vi "Process.vi"(8 "error in":errorcluster, 11 "Instrument.Transport in":refnum<class "Inst.Transport.lvclass">) -> (0 "error out":errorcluster, 3 "Instrument.Transport out":refnum<class "Inst.Transport.lvclass">)   [LabVIEW 2019, in "Inst.Transport.lvclass"]
doc: "---------------------------------------------------------------\nJKI State Machine Objects™\nhttp://jki.net/state-machine-objects/\nCopyright (C) 2005-2015, JKI <info@jki.net>\nALL RIGHTS RESERVED"
uses:
  Inst.Transport.lvclass
  <userlib>/LevyLab/Instrument Framework/Instrument/Instrument.lvclass
  <userlib>/LevyLab/RemoteControl/RemoteControl/Typedefs/Message--Cluster.ctl
  <userlib>/LevyLab/RemoteControl/RemoteControl/RemoteControl.lvclass
  Typedefs/PrivateEvents--MessageToProcess.ctl
  <userlib>/LevyLab/Debug/Debug.lvlib
  <vilib>/JKI/JKI SMO/SMO/SMO.lvclass
  <userlib>/LevyLab/Instrument Framework/Instrument Types/SCPI/Instrument.SCPI.lvclass
  <userlib>/LevyLab/Transport/Control Experiment/Control Experiment.lvclass
  <userlib>/LevyLab/Transport/Transport/Transport.lvclass
  <vilib>/platform/TimedLoop/XDataNode/XDataNode.xnode
  <vilib>/Platform/TimedLoop/XDataNode/timing_clust.ctl
  <vilib>/Platform/TimedLoop/XDataNode/XDNodeRunTimeDep.lvlib
  <vilib>/Platform/TimedLoop/XDataNode/wakeup.ctl
  <vilib>/Platform/TimedLoop/XDataNode/nitl_modes.ctl
  <userlib>/LevyLab/Lockin-Multichannel/Instrument.DAQ/Typedefs/Sweep.Pattern--Enum.ctl
  <userlib>/LevyLab/Lockin-Multichannel/Instrument.DAQ/Instrument.DAQ.lvclass
  <userlib>/LevyLab/Lockin-Multichannel/Instrument.DAQ/Typedefs/Sweep.Channel--Cluster.ctl
  <userlib>/LevyLab/Lockin-Multichannel/Instrument.DAQ/Typedefs/Sweep.Channel--Cluster--Array.ctl
  <userlib>/LevyLab/Transport/Transport/Typedefs/Lockin_Sweep JSON--Cluster.ctl
  <userlib>/LevyLab/Instrument Framework/Instrument/API/Instrument.sendMessageToProcess (variant).vi
  C:/Program Files (x86)/National Instruments/LabVIEW 2019/user.lib/LevyLab/Instrument Framework/Instrument Types/SCPI/Instrument.SCPI.lvclass
  C:/Program Files (x86)/National Instruments/LabVIEW 2019/user.lib/LevyLab/Instrument Framework/Instrument/Instrument.lvclass
  C:/Program Files (x86)/National Instruments/LabVIEW 2019/vi.lib/JKI/JKI SMO/SMO/SMO.lvclass
panel:
  in  "stop 2":bool
  in  "stop":bool
  out "Calling VI":string
  out "Experiment Folder":string
  out "Comments":string
  out "TDMS Params":cluster{"Key":string, "Value":dbl}[](array[cluster])
  out "Status":string
  out "State History":string
  # "Instrument.Framework-Template"
  # "Framework-Template"
  # "For instructions on how to use the JKI State Machine Objects, examples and video tutorials, visit:\nhttp://jki.net/state-machine-objects/\n\nJKI State Machine Objects™\nhttp://jki.net/state-machine-objects/\nCopyright (C) 2005-2015, JKI <info@jki.net>\nALL RIGHTS RESERVED"
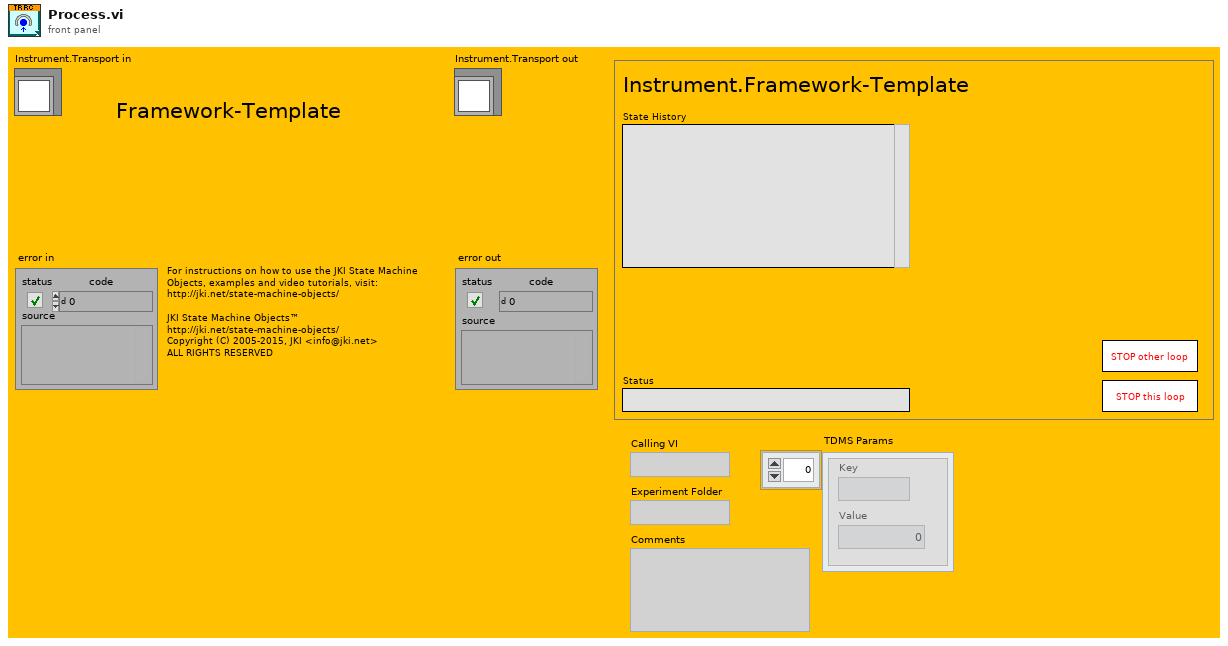
[diagram p1: front panel]
types:
  T1 = typedef "Transport.lvclass/Lockin_Sweep JSON--Cluster.ctl" = cluster{"Sweep Time (s)":dbl, "Initial Wait (s)":dbl, "Return to Start":bool, "Sweep Channels":T2, "Sweep Tables":cluster{"Ch":i32, "Table":dbl[]}[]}
  T2 = typedef "Instrument.Lockin.lvlib/Instrument.DAQ.lvclass/Sweep.Channel--Cluster--Array.ctl" = T3[]
  T3 = typedef "Instrument.Lockin.lvlib/Instrument.DAQ.lvclass/Sweep.Channel--Cluster.ctl" = cluster{"Enable?":bool, "Channel":u16, "Start":dbl, "End":dbl, "Pattern":T4, "Table":dbl[]}
  T4 = typedef "Instrument.Lockin.lvlib/Instrument.DAQ.lvclass/Sweep.Pattern--Enum.ctl" = enum16{"Ramp /", "Ramp /\\", "Smooth Ramp _/", "Smooth Ramp _/\\_", "Table"}
  T5 = enum32{"invalid app kind", "Development System", "Run Time System", "Student Edition", "Embedded LabVIEW", "Evaluation", "Custom"}
  T6 = enum32{"Invalid", "Standard", "Closed", "Hidden", "Minimized", "Maximized"}
  T7 = typedef "RemoteControl.lvlib/RemoteControl.lvclass/Message--Cluster.ctl" = cluster{"Command":string, "Data":variant, "ID":string}
  T8 = typedef "Inst.Transport.lvclass/PrivateEvents--MessageToProcess.ctl" = cluster{"Message":T7}
  T9 = cluster{"Core":cluster{"Current VI Reference":refnum<vi>, "Close Panel on Exit?":bool, "Last Error":cluster{"error":errorcluster, "previous state":string, "remaining states":string}, "Shutdown?":bool}, "SelfRef":refnum<class "Inst.Transport.lvclass">, "HAL":refnum<class "HAL.lvclass">, "Running Step":i32, "sequence":string[], "MessageToProcess":T8, "UI Behavior":string, "wait":u32}
  T10 = cluster{"Current VI Reference":refnum<vi>, "Close Panel on Exit?":bool, "Last Error":cluster{"error":errorcluster, "previous state":string, "remaining states":string}, "Shutdown?":bool}
  T11 = typedef "Debug.lvlib/Attribute.Debug.lvclass/DebugBehavior.ctl" = enum16{"Normal", "Debug"}
  T12 = typedef "SMO.lvclass/Protected Events.ctl" = cluster{"StopProcesses":refnum<user-event>, "AbortProcesses":refnum<user-event>, "Config Changed":refnum<user-event>, "Dependency":refnum<user-event>}
  T13 = typedef "Inst.Transport.lvclass/Inst.Transport.getAll--Cluster.ctl" = cluster{"Levy 1":dbl, "Logger SMO":dbl, "SMO Boolean":bool, "SMO String":string}
  T14 = typedef "XDNodeRunTimeDep.lvlib/timing_clust.ctl" = cluster{"Expected End [f-1]":u64, "Actual End [f-1]":u64, "Finished Late? [f-1]":bool, "Expected End [i-1]":u64, "Actual End [i-1]":u64, "Finished Late? [i-1]":bool, "Expected Start [i]":u64, "Actual Start [i]":u64, "Expected Start [f]":u64, "Actual Start [f]":u64, "Source Name":string, "Structure Name":string, "Period":i64, "Deadline":i64, "Offset":i64, "Start":i64, "Priority":i32, "Timeout":i32, "Mode":T15, "Wakeup Reason":T16, "Error":errorcluster, "Source Type":string, "Secondary Source Type":string, "Global End Time":u64, "Global Start Time":u64, "Frame Duration":u64, "Iteration Duration":u64, "Assigned CPU":i32, "I/O Scan Engine Mode":u32}
  T15 = typedef "XDNodeRunTimeDep.lvlib/nitl_modes.ctl" = enum32{"No Change", "Process missed periods, maintain original phase", "Discard missed periods, maintain original phase", "Process missed periods, ignore original phase", "Discard missed periods, ignore original phase"}
  T16 = typedef "XDNodeRunTimeDep.lvlib/wakeup.ctl" = enum32{"Normal", "Aborted", "Asynchronous wakeup", "Timing source error", "Timed loop error", "Timeout"}
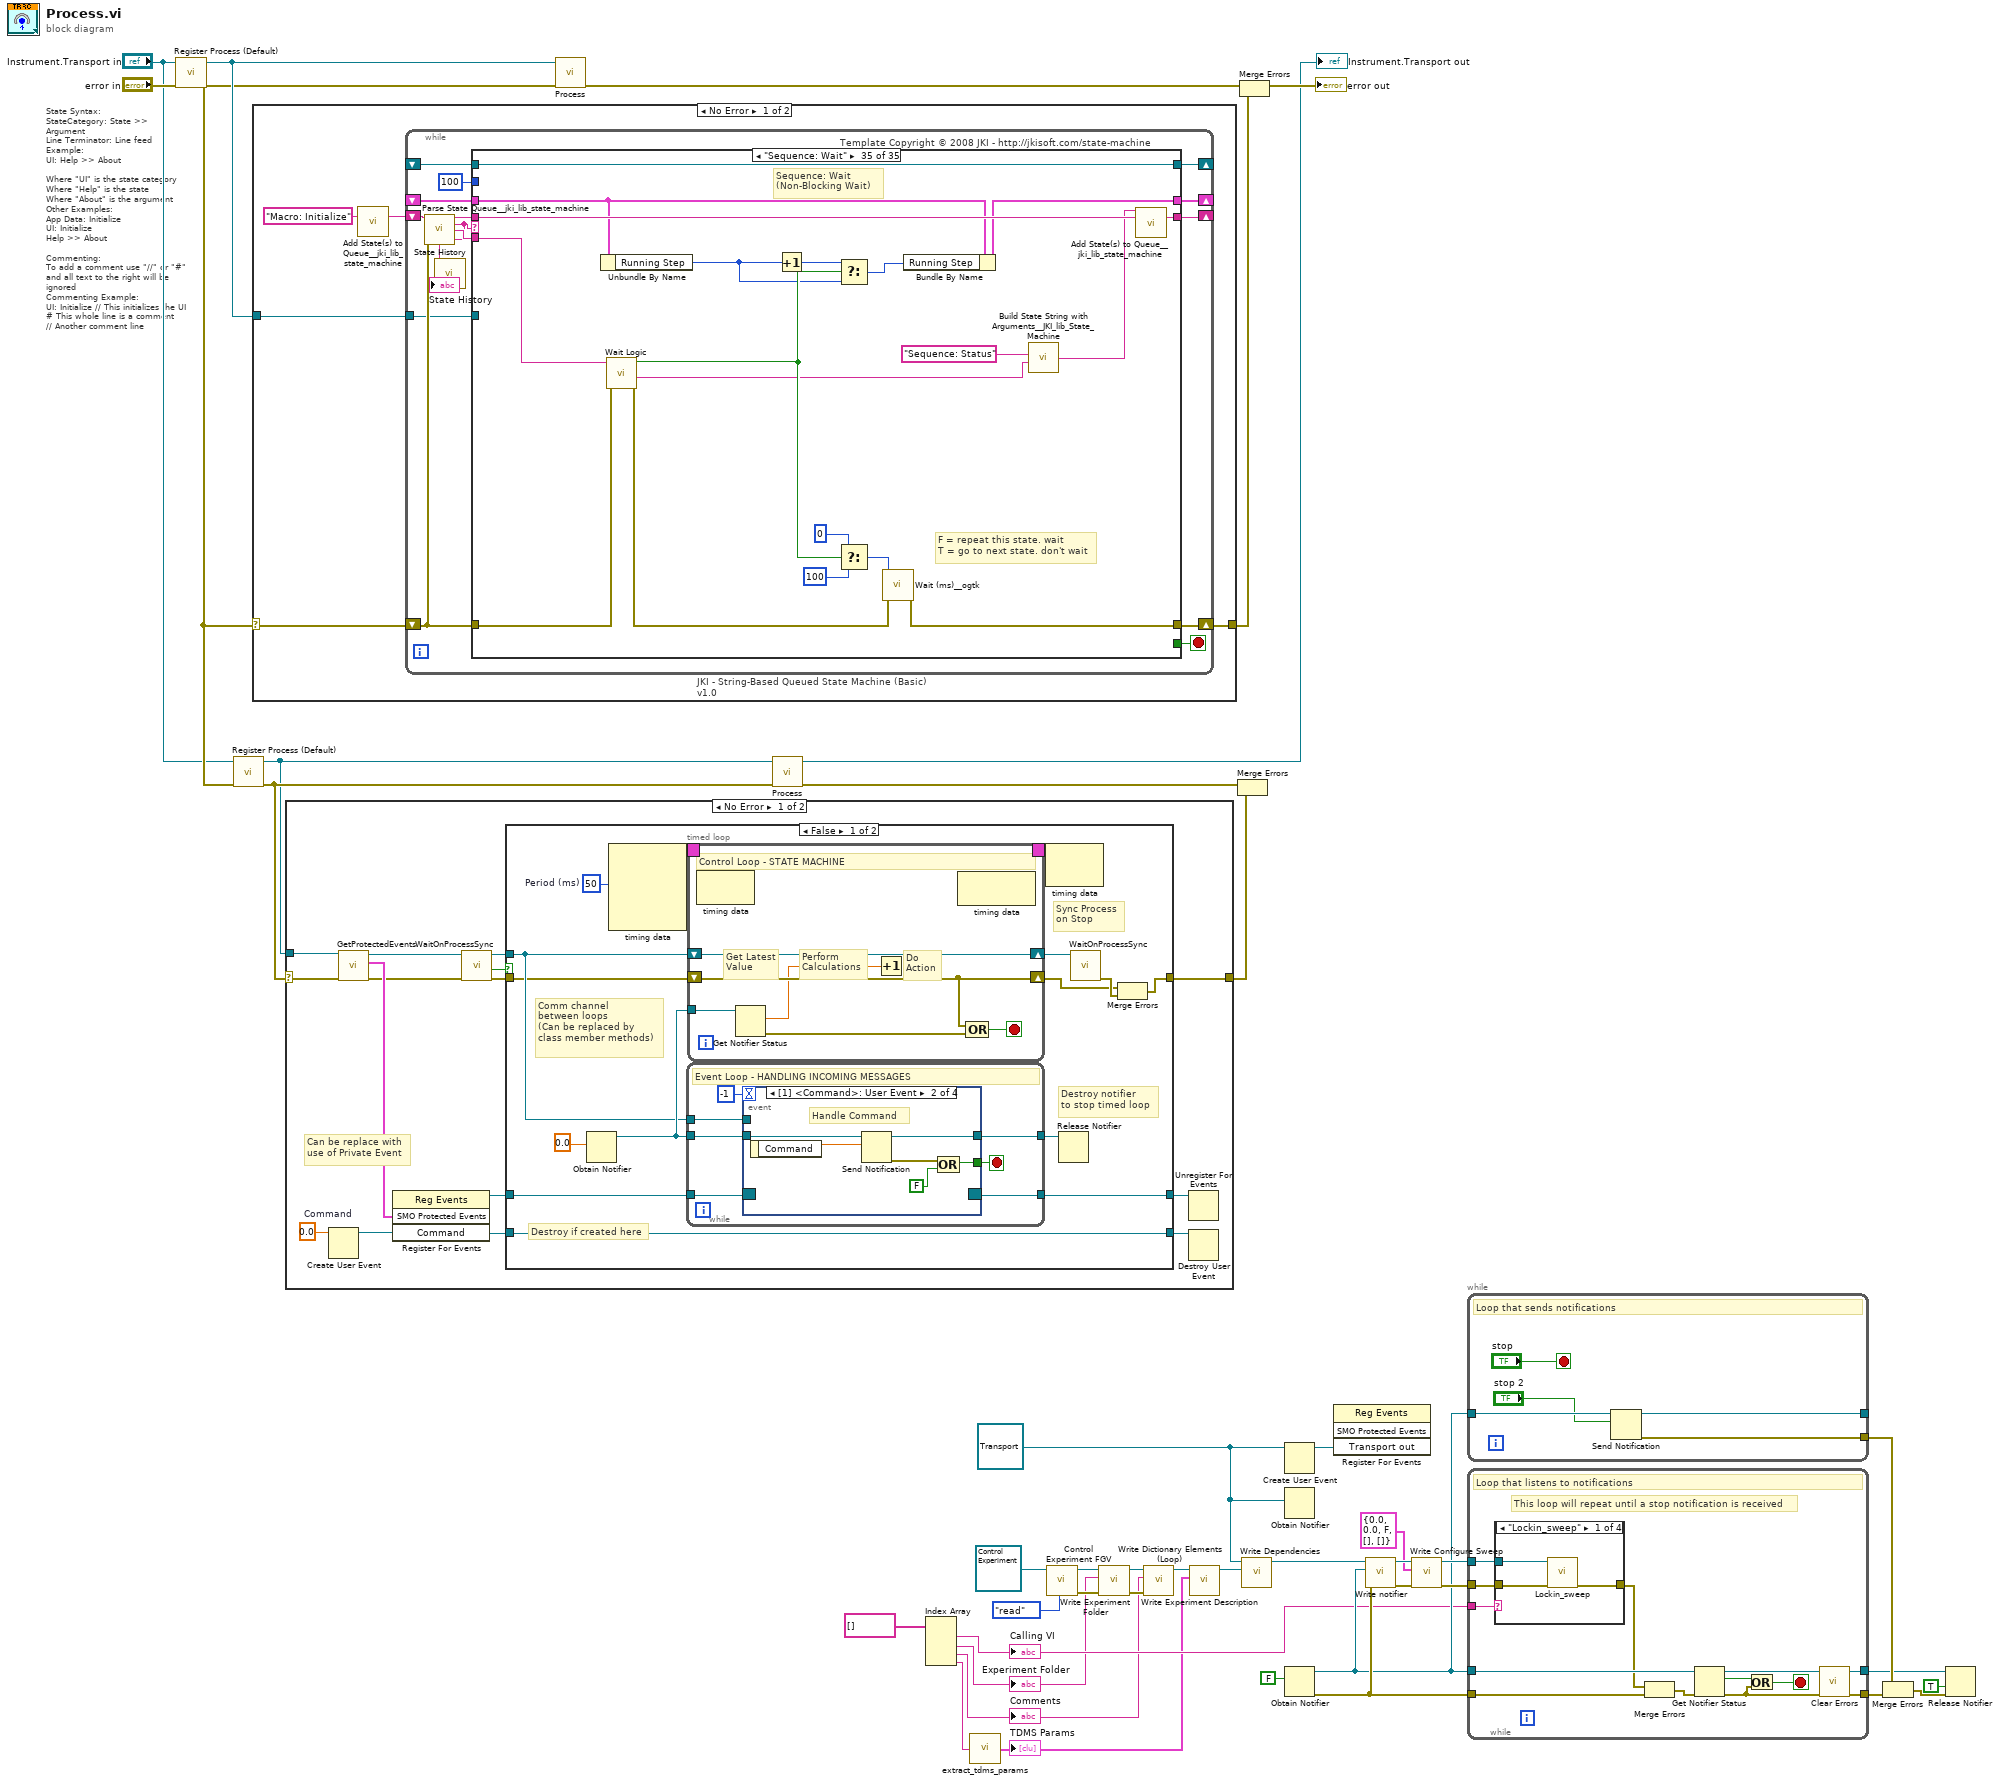
[diagram p0: block diagram]
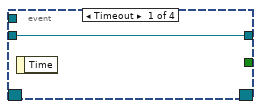
[diagram p2: hidden frame]
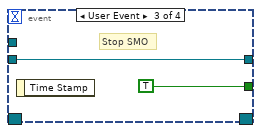
[diagram p3: hidden frame]
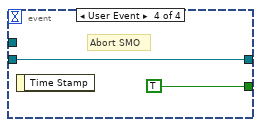
[diagram p4: hidden frame]
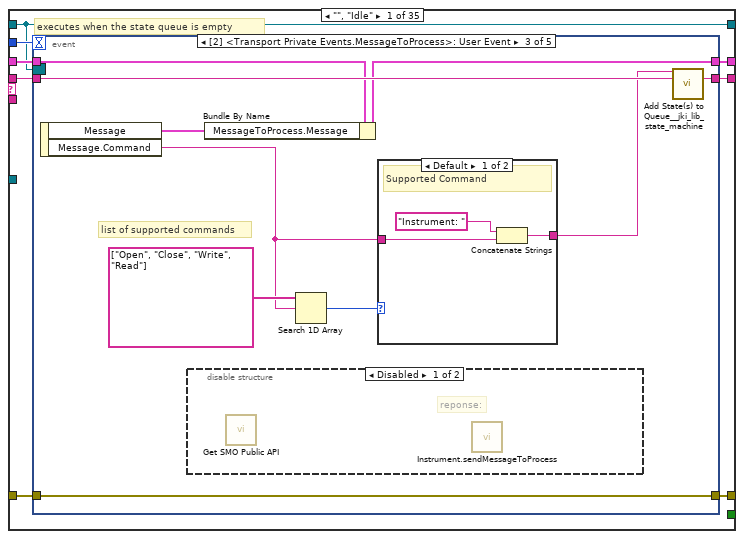
[diagram p7: hidden frame]
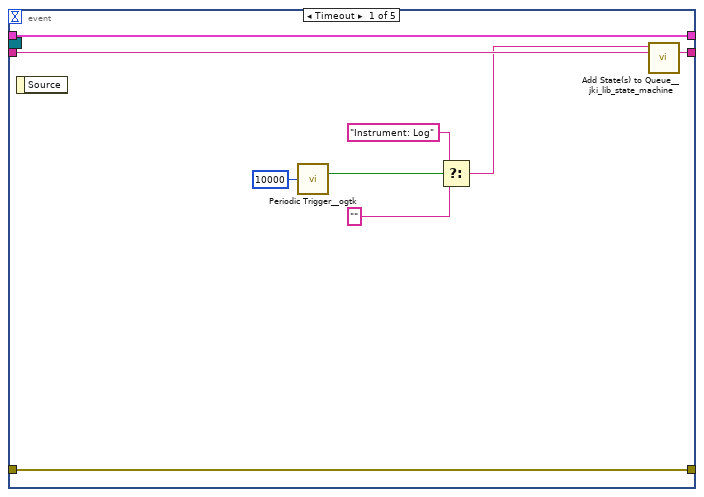
[diagram p8: hidden frame]
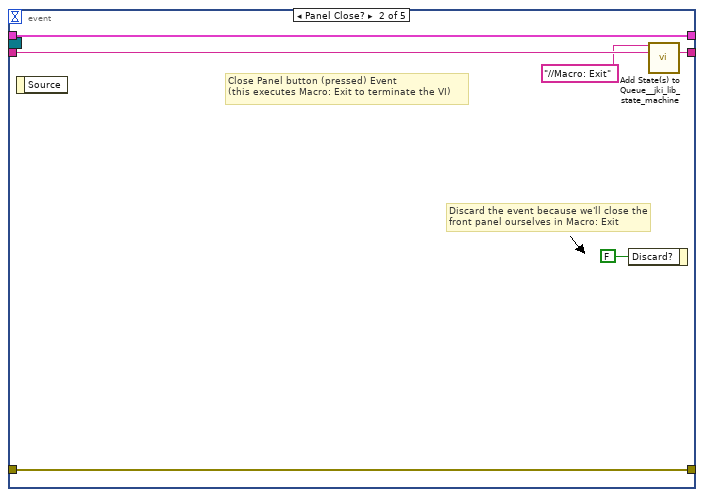
[diagram p9: hidden frame]
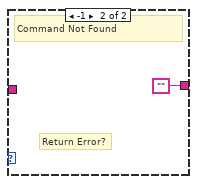
[diagram p11: hidden frame]
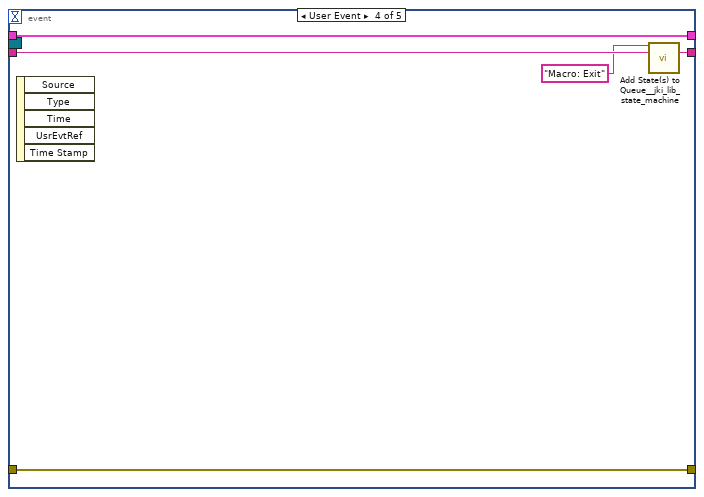
[diagram p12: hidden frame]
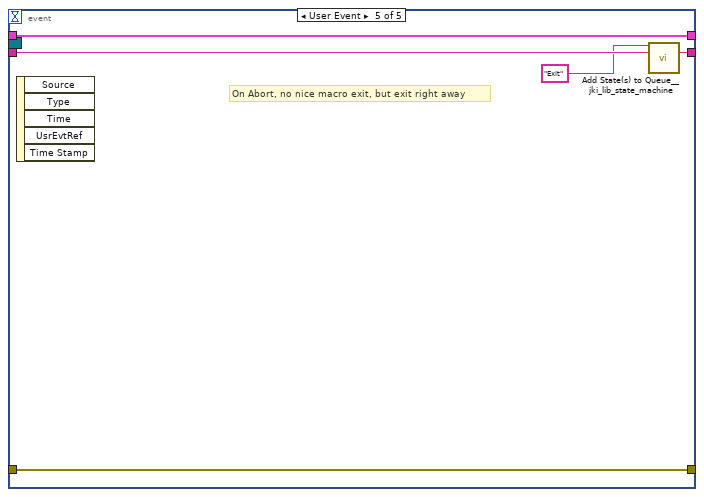
[diagram p13: hidden frame]
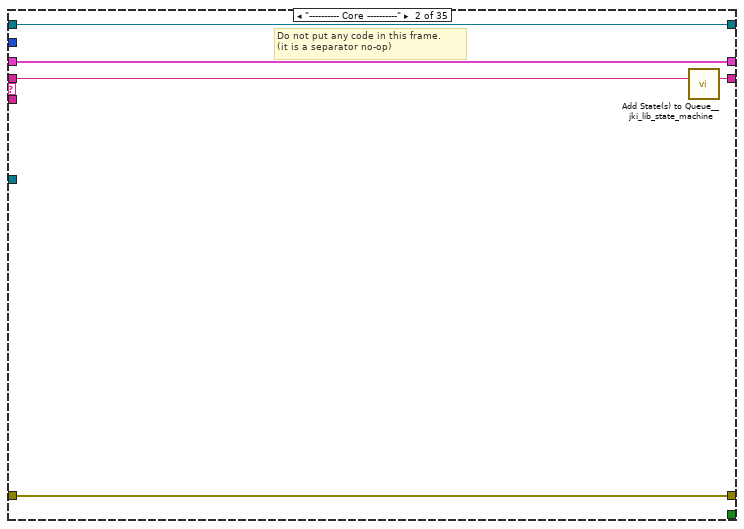
[diagram p14: hidden frame]
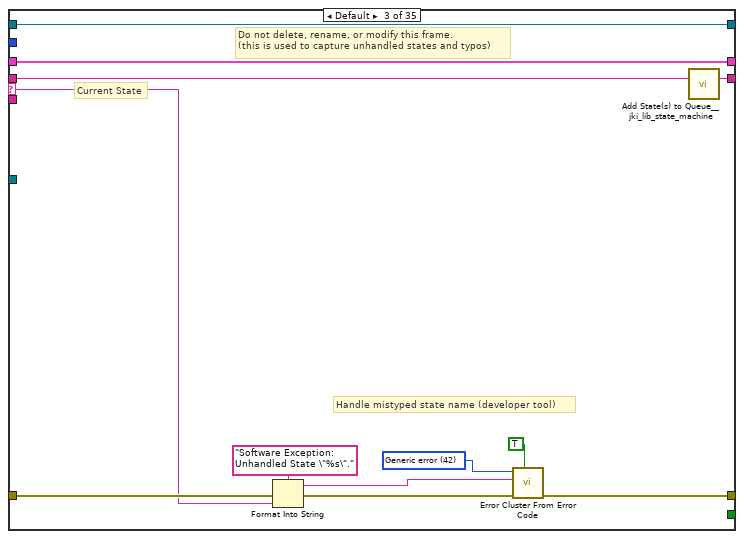
[diagram p15: hidden frame]
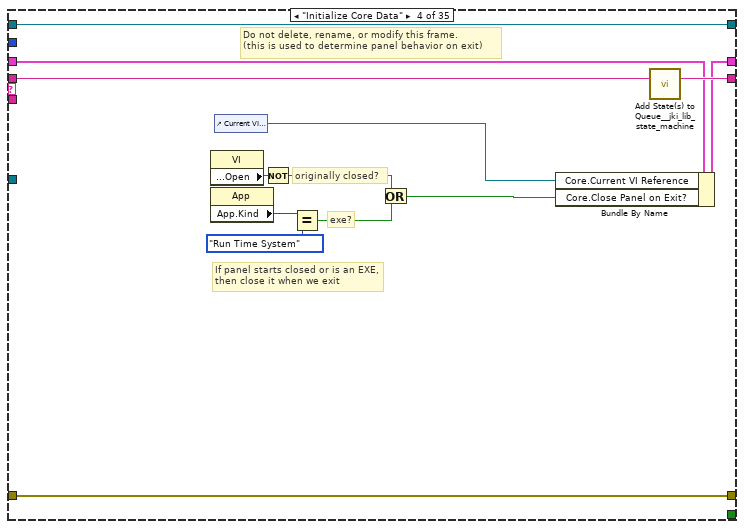
[diagram p16: hidden frame]
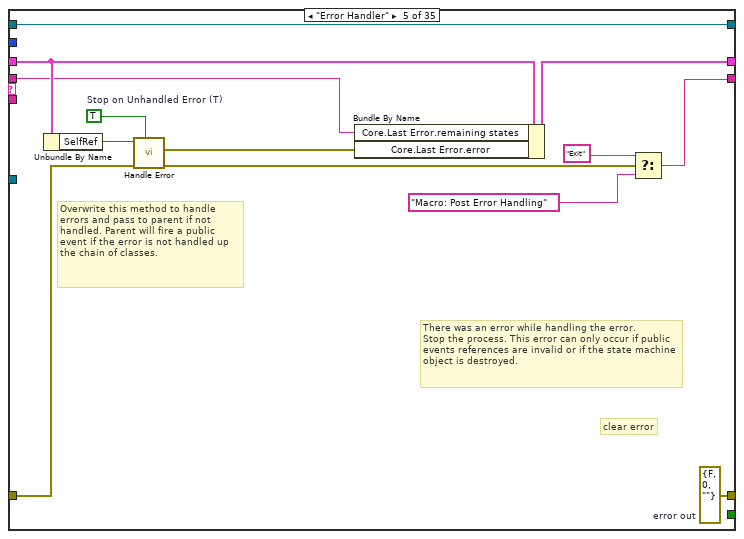
[diagram p17: hidden frame]
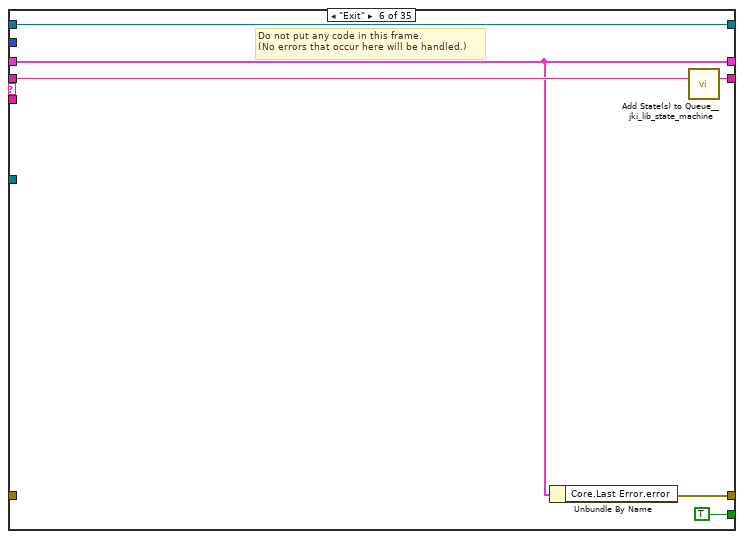
[diagram p18: hidden frame]
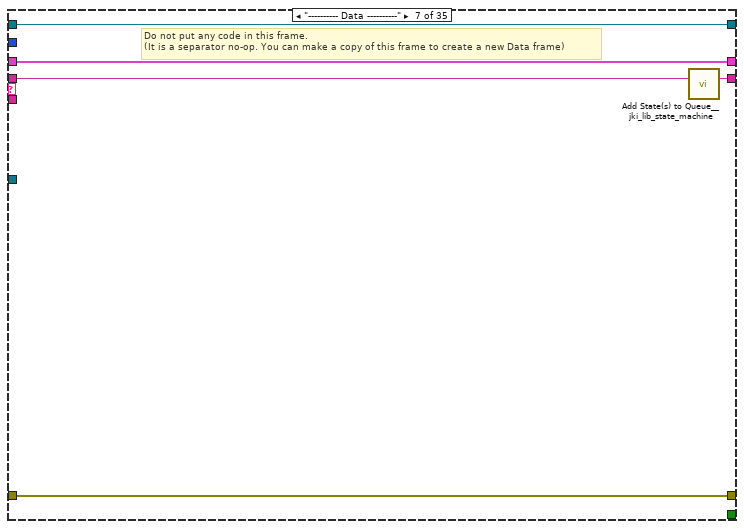
[diagram p19: hidden frame]
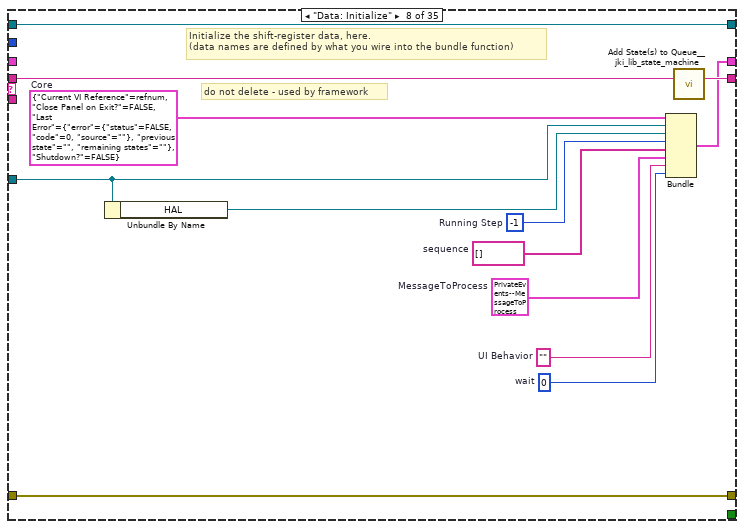
[diagram p20: hidden frame]
diagram:
  w2 = refnum<class "Transport.lvclass"> refnum ("Transport out")
  # "State Syntax:\nStateCategory: State >> Argument\nLine Terminator: Line feed\nExample:\nUI: Help >> About\n\nWhere \"UI\" is the state category\nWhere \"Help\" is the state\nWhere \"About\" is the argument\nOther Examples:\nApp Data: Initialize\nUI: Initialize\nHelp >> About\n\nCommenting:\nTo add a comment use \"//\" or \"#\" and all text to the right will be ignored\nCommenting Example:\nUI: Initialize // This initializes the UI\n# This whole line is a comment\n// Another comment line"
  n1 = call <vilib>:"Register Process (Default).vi"("error in (no error)"="error in", "SMO"="Instrument.Transport in") -> ("error out"=w33:errorcluster, "SelfRef"=w40:refnum<class "Inst.Transport.lvclass">)  [unwired: 8 in]
  n2 = call <vilib>:"Register Process (Default).vi"("error in (no error)"=w33, "SMO"="Instrument.Transport in") -> ("error out"=w37:errorcluster, "SelfRef"=w36:refnum<class "Inst.Transport.lvclass">)  [unwired: 8 in]
  n3 = case shown="No Error" w33 {
    selector: w33 -> [w44 w486]
    tunnel: w40 -> [w45 _]
    tunnel: [w43 w486] -> w38
    frame No Error {
      n4 = call <vilib>:"Add State(s) to Queue__jki_lib_state_machine.vi"("State(s) in (\"\")"="Macro: Initialize") -> ("States Out"=w47:string)  [unwired: 14 in]
      n5 = while "JKI - String-Based Queued State Machine (Basic) v1.0" {
        shift-right: [w56] -> _
        shift-left: _ -> [w55]
        shift-right: [w59] -> w43
        shift-left: w44 -> [w53]
        shift-right: [w58] -> _
        shift-left: w47 -> [w60]
        tunnel: w45 -> [w52]
        shift-right: [w51] -> _
        shift-left: _ -> [w50]
        stop <- w57 stop-if-true
        # "Template Copyright © 2008 JKI - http://jkisoft.com/state-machine"
        n6 = call <vilib>:"Parse State Queue__jki_lib_state_machine.vi"("State Queue"=w60, "Error In (no error)"=w53) -> ("Remaining States"=w62:string, "Current State"=w49:string, "Arguments"=w61:string)  [unwired: 11 in]
        n7 = call <userlib>:"State History.vi"("Current State"=w49) -> ("History"=→"State History":string)  [unwired: 10 in]
        n8 = case shown="\"Sequence: Wait\"" w49 {
          selector: w49 -> [_ _ w116 _ _ _ _ _ _ _ _ _ _ _ _ _ _ _ _ _ _ _ _ _ _ _ _ _ _ _ _ _ _ _ _]
          tunnel: w62 -> [w70 w114 w120 w139 w144 w158 w163 w176 w183 w188 w195 w204 w211 w227 w259 w268 w280 w301 w316 w338 w343 w354 w359 w372 w378 w386 w395 w404 w414 w423 w435 w455 w460 w466 w485]
          tunnel: w61 -> [_ _ _ _ _ _ _ _ _ _ _ w196 w205 w221 _ _ _ _ _ _ _ _ _ _ _ _ _ _ _ _ _ _ _ w461 w469]
          tunnel: w55 -> [w68 w111 w118 w130 w148 w154 w160 _ w178 w185 w193 w201 w209 w223 w256 w265 w270 w291 w305 w323 w340 w351 w356 w365 w376 w381 w391 w400 w410 w419 w431 w451 w456 w462 w475]
          tunnel: [w67 w112 w122 w136 w149 w153 w161 w166 w179 w186 w190 w202 w206 w224 w257 w260 w278 w299 w304 w326 w341 w345 w357 w368 w374 w383 w387 w399 w409 w418 w426 w449 w457 w463 w477] -> w59
          tunnel: w53 -> [w66 w112 w121 w136 w150 _ w161 w166 w180 w186 w189 w202 w207 w225 w257 w260 w278 w299 w303 w326 w341 w346 w357 w362 w374 w383 w390 w398 w408 w417 w429 w444 w457 w463 w471]
          tunnel: [w69 w113 w119 w138 w140 w157 w162 w175 w182 w187 w194 w203 w210 w226 w258 w267 w279 w300 w315 w337 w342 w353 w358 w371 w377 w385 w394 w403 w413 w422 w434 w454 w459 w465 w484] -> w58
          tunnel: [_ _ _ _ _ TRUE _ _ _ _ _ _ _ _ _ _ _ _ _ _ _ _ _ _ _ _ _ _ _ _ _ _ _ _ _] -> w57
          tunnel: [w65 w111 w118 w137 w147 w154 w160 w174 w178 w185 w193 w201 w209 w223 w256 w265 w271 w292 w306 w324 w340 w351 w356 w365 w376 w382 w392 w401 w411 w420 w432 w452 w456 w462 w474] -> w56
          tunnel: 100 ("Timeout") -> [w64 _ _ _ _ _ _ _ _ _ _ _ _ _ _ _ _ _ _ _ _ _ _ _ _ _ _ _ _ _ _ _ _ _ _]
          tunnel: w52 -> [_ _ _ _ _ _ _ w167 _ _ _ _ _ _ _ _ _ _ _ _ _ _ _ _ _ _ _ _ _ _ _ _ _ _ _]
          tunnel: [w63 w110 w115 w127 w152 w155 w159 w173 w177 w184 w192 w200 w208 w220 w255 w266 w277 w298 w314 w332 w339 w352 w355 w370 w375 w384 w393 w402 w412 w421 w433 w453 w458 w464 w483] -> w51
          tunnel: w50 -> [w63 w110 w115 w127 w152 w155 w159 w173 w177 w184 w192 w200 w208 w220 w255 w266 w277 w298 w314 w332 w339 w352 w355 _ w375 w384 w393 w402 w412 w421 w433 w453 w458 w464 w483]
          frame "", "Idle" {
            # "executes when the state queue is empty"
            n9 = event shown="[2] <Transport Private Events.MessageToProcess>: User Event" {
              selector: w63 -> [_ _ _ _ _]
              dyn-events: _ -> [_ _ _ _ _]
              timeout: w64 -> [_ _ _ _ _]
              tunnel: w70 -> [w79 w85 w95 w104 w109]
              tunnel: [w78 w84 w94 w103 w108] -> w69
              tunnel: w68 -> [w76 w82 w87 w101 w106]
              tunnel: [w77 w83 w93 w102 w107] -> w67
              tunnel: w66 -> [w77 w83 w93 w102 w107]
              tunnel: [w76 w82 w88 w101 w106] -> w65
              event Timeout {
                n10 = event-data() -> ()  [unwired: 1 in, 1 out]
                n11 = call <userlib>:"Periodic Trigger__ogtk.vi"("time (ms)"=u32 10000) -> ("Triggered"=w73:bool)  [unwired: 12 in, 2 out]
                n12 = Select(t="Instrument: Log", s=w73, f="") -> (s? t:f=w74:string)
                n13 = call <vilib>:"Add State(s) to Queue__jki_lib_state_machine.vi"("State(s) in Front (\"\")"=w74, "State(s) in (\"\")"=w79) -> ("States Out"=w78:string)  [unwired: 13 in]
              }
              event Panel Close? {
                # "Discard the event because we'll close the front panel ourselves in Macro: Exit"
                # "Close Panel button (pressed) Event\n(this executes Macro: Exit to terminate the VI)"
                n14 = event-data() -> ()  [unwired: 1 in, 1 out]
                n15 = event-data("Discard?"=FALSE) -> ()  [unwired: 1 in, 1 out]
                n16 = call <vilib>:"Add State(s) to Queue__jki_lib_state_machine.vi"("State(s) in Front (\"\")"="//Macro: Exit", "State(s) in (\"\")"=w85) -> ("States Out"=w84:string)  [unwired: 13 in]
              }
              event User Event {
                # "list of supported commands"
                n17 = event-data() -> ("Message"=w86:T7, "Message.Command"=w89:string)  [unwired: 1 in]
                n18 = disable-structure shown="Disabled" {
                  frame Disabled {
                    # "reponse:"
                    n19 = call-dynamic "Get SMO Public API.vi"() -> ()  [unwired: 9 in, 3 out]
                    n20 = call-poly <userlib>:"Instrument.sendMessageToProcess.vi"() -> ()  [unwired: 10 in, 2 out]
                  }
                  frame Enabled {
                  }
                }
                n21 = Bundle By Name(cluster=w87, "MessageToProcess.Message"=w86) -> (w88:T9)
                n22 = Search 1D Array(1D array=string[] ["Open", "Close", "Write", "Read"], element=w89) -> (index of element=w92:i32)  [unwired: 1 in]
                n23 = case shown="Default" w92 {
                  tunnel: [w98 "" ("Empty String Constant")] -> w90
                  tunnel: w89 -> [w97 _]
                  frame Default {
                    # "Supported Command"
                    n24 = Concatenate Strings("Instrument: ", w97) -> (w98:string)
                  }
                  frame -1 {
                    # "Return Error?"
                    # "Command Not Found"
                  }
                }
                n25 = call <vilib>:"Add State(s) to Queue__jki_lib_state_machine.vi"("State(s) in Front (\"\")"=w90, "State(s) in (\"\")"=w95) -> ("States Out"=w94:string)  [unwired: 13 in]
              }
              event User Event {
                n26 = event-data() -> ()  [unwired: 1 in, 5 out]
                n27 = call <vilib>:"Add State(s) to Queue__jki_lib_state_machine.vi"("State(s) in Front (\"\")"="Macro: Exit", "State(s) in (\"\")"=w104) -> ("States Out"=w103:string)  [unwired: 13 in]
              }
              event User Event {
                # "On Abort, no nice macro exit, but exit right away"
                n28 = event-data() -> ()  [unwired: 1 in, 5 out]
                n29 = call <vilib>:"Add State(s) to Queue__jki_lib_state_machine.vi"("State(s) in Front (\"\")"="Exit", "State(s) in (\"\")"=w109) -> ("States Out"=w108:string)  [unwired: 13 in]
              }
            }
          }
          frame "---------- Core ----------" {
            # "Do not put any code in this frame.\n(it is a separator no-op)"
            n30 = call <vilib>:"Add State(s) to Queue__jki_lib_state_machine.vi"("State(s) in (\"\")"=w114) -> ("States Out"=w113:string)  [unwired: 14 in]
          }
          frame Default {
            w125 = 42 items=["No error", "Argument error", "Memory is full", "Out of zone", "End of file", "File already open", "Generic file I/O error", "File not found", "File permission error", "Disk is full", "Duplicate path", "Too many files open", "System feature not enabled", "Resource file not found", "Cannot add resource", "Resource not found", "Image not found", "Image memory error", "Pen does not exist", "Config type invalid", "Config token not found", "Config parse error", "Config memory error", "Bad external code format", "Bad external code offset", "External code not present", "Null window", "Destroy window error", "Null menu", "Print aborted", "Bad print record", "Print driver error", "Windows error during printing", "Memory error during printing", "Print dialog error", "Generic print error", "Invalid device refnum", "Device not found", "Device parameter error", "Device unit error", "Cannot open device", "Device call aborted", "Generic error", "Cancelled by user", "Object ID too low", "Object ID too high", "Object not in heap", "Unknown heap", "Unknown object (invalid DefProc)", "Unknown object (DefProc not in table)", "Message out of range", "Invalid (null) method", "Unknown message", "Manager call not supported", "Bad address", "Network operation in progress", "Network operation timed out", "Connection is busy", "Network attribute not supported", "Network error", "Address in use", "System out of memory", "Connection aborted", "Connection refused", "Not connected", "Already connected", "Connection closed", "Initialization error (interapplication manager)", "Bad occurrence", "Wait on unbound occurrence handler", "Occurrence queue overflow", "Datalog type conflict", "Unused", "Unrecognized type (interapplication manager)", "Memory corrupt", "Failed to make temporary DLL", "Old CIN version", "Drag socket not found", "Failed to load drop-object", "Failed to register OLE object", "Failed to release OLE object", "Format specifier type mismatch", "Unknown format specifier", "Too few format specifiers", "Too many format specifiers", "Scan failed", "Newer CIN version", "Error converting to variant", "Runtime menu error", "Password tampered", "Variant attribute not found", "Incompatible variant data type", "Event data is not available", "Event Store is not present", "Occurrence is not found", "Event Queue is not created", "Event info is not available", "Refnum passed is NULL", "Error retrieving Class GUID", "Error retrieving CoClass GUID", "Error retrieving TypeLib GUID.", "Bad built application magic bytes.", "Specific driver is different from the specific driver associated with the Logical Name.", "There is no session opened to the class driver.", "Max Error", "MAX - Error with config objects", "MAX - Error loading configuration", "MAX - Group not supported"]
            # "Current State"
            # "Do not delete, rename, or modify this frame.\n(this is used to capture unhandled states and typos)"
            # "Handle mistyped state name (developer tool)"
            n31 = Format Into String(format string="Software Exception: Unhandled State \"%s\"." ("message"), error in=w121, w116) -> (resulting string=w124:string, error out=w123:errorcluster)  [unwired: 1 in]
            n32 = call <vilib>:"Error Cluster From Error Code.vi"("show call chain? (False)"=TRUE, "error in (no error)"=w123, "error message (\"\")"=w124, "error code (0)"=w125) -> ("error out"=w122:errorcluster)  [unwired: 5 in]
            n33 = call <vilib>:"Add State(s) to Queue__jki_lib_state_machine.vi"("State(s) in (\"\")"=w120) -> ("States Out"=w119:string)  [unwired: 14 in]
          }
          frame "Initialize Core Data" {
            # "Do not delete, rename, or modify this frame.\n(this is used to determine panel behavior on exit)"
            # "originally closed?"
            # "exe?"
            # "If panel starts closed or is an EXE, then close it when we exit"
            n34 = property class="VI"() -> ("Front Panel.Open"=w135:bool)  [unwired: 2 in, 2 out]
            n35 = property class="App"() -> ("App.Kind"=w134:T5)  [unwired: 2 in, 2 out]
            n36 = control-ref of="Current VI Reference"() -> (w128:refnum<vi>)
            n37 = Not(x=w135) -> (.not. x?=w132:bool)
            n38 = Equal?(x=w134, y=T5."Run Time System" ("Application:Kind")) -> (x = y?=w131:bool)
            n39 = Or(x=w132, y=w131) -> (x .or. y?=w129:bool)
            n40 = Bundle By Name(cluster=w130, "Core.Current VI Reference"=w128, "Core.Close Panel on Exit?"=w129) -> (w137:T9)
            n41 = call <vilib>:"Add State(s) to Queue__jki_lib_state_machine.vi"("State(s) in (\"\")"=w139) -> ("States Out"=w138:string)  [unwired: 14 in]
          }
          frame "Error Handler" {
            w145 = TRUE  # Stop on Unhandled Error (T)
            w149 = errorcluster {"status"=FALSE, "code"=0, "source"=""}  # error out
            # "clear error"
            # "There was an error while handling the error.\nStop the process. This error can only occur if public events references are invalid or if the state machine object is destroyed."
            # "Overwrite this method to handle errors and pass to parent if not handled. Parent will fire a public event if the error is not handled up the chain of classes."
            n42 = Unbundle By Name(w148) -> ("SelfRef"=w151:refnum<class "Inst.Transport.lvclass">)
            n43 = call-dynamic "Handle Error.vi"("Stop on Unhandled Error (T)"=w145, "error in"=w150, "SMO"=w151) -> ("handling error"=w141:errorcluster, "Unhandled error"=w146:errorcluster)  [unwired: 6 in, 1 out]
            n44 = Bundle By Name(cluster=w148, "Core.Last Error.remaining states"=w144, "Core.Last Error.error"=w146) -> (w147:T9)
            n45 = Select(t="Exit", s=w141, f="Macro: Post Error Handling") -> (s? t:f=w140:string)
          }
          frame "Exit" {
            # "Do not put any code in this frame.\n(No errors that occur here will be handled.)"
            n46 = Unbundle By Name(w154) -> ("Core.Last Error.error"=w153:errorcluster)
            n47 = call <vilib>:"Add State(s) to Queue__jki_lib_state_machine.vi"("State(s) in (\"\")"=w158) -> ("States Out"=w157:string)  [unwired: 14 in]
          }
          frame "---------- Data ----------" {
            # "Do not put any code in this frame.\n(It is a separator no-op. You can make a copy of this frame to create a new Data frame)"
            n48 = call <vilib>:"Add State(s) to Queue__jki_lib_state_machine.vi"("State(s) in (\"\")"=w163) -> ("States Out"=w162:string)  [unwired: 14 in]
          }
          frame "Data: Initialize" {
            w164 = u32 0  # wait
            w165 = ""  # UI Behavior
            w169 = T8 {"Message"={"Command"="", "Data"=variant(string ""), "ID"=""}}  # MessageToProcess
            w170 = string[] []  # sequence
            w171 = -1  # Running Step
            w172 = T10 {"Current VI Reference"=refnum, "Close Panel on Exit?"=FALSE, "Last Error"={"error"={"status"=FALSE, "code"=0, "source"=""}, "previous state"="", "remaining states"=""}, "Shutdown?"=FALSE}  # Core
            # "do not delete - used by framework"
            # "Initialize the shift-register data, here.\n(data names are defined by what you wire into the bundle function)"
            n49 = Unbundle By Name(w167) -> ("HAL"=w168:refnum<class "HAL.lvclass">)
            n50 = Bundle("Core"=w172, "SelfRef"=w167, "HAL"=w168, "Running Step"=w171, "sequence"=w170, "MessageToProcess"=w169, "UI Behavior"=w165, "wait"=w164) -> (w174:T9)  [unwired: 1 in]
            n51 = call <vilib>:"Add State(s) to Queue__jki_lib_state_machine.vi"("State(s) in (\"\")"=w176) -> ("States Out"=w175:string)  [unwired: 14 in]
          }
          frame "Data: Cleanup" {
            # "Cleanup any data and references, here.\n(this is called automatically, by the Macro: Exit)"
            n52 = Unbundle By Name(w178) -> ("Core.Current VI Reference"=w181:refnum<vi>)
            n53 = Close Reference(reference=w181, error in (no error)=w180) -> (error out=w179:errorcluster)
            n54 = call <vilib>:"Add State(s) to Queue__jki_lib_state_machine.vi"("State(s) in (\"\")"=w183) -> ("States Out"=w182:string)  [unwired: 14 in]
          }
          frame "---------- UI ----------" {
            # "Do not put any code in this frame.\n(It is a separator no-op. You can make a copy of this frame to create a new UI frame)"
            n55 = call <vilib>:"Add State(s) to Queue__jki_lib_state_machine.vi"("State(s) in (\"\")"=w188) -> ("States Out"=w187:string)  [unwired: 14 in]
          }
          frame "UI: Initialize" {
            # "Initialize the User Interface, here.\n(this is called automatically, by the Macro: Init)"
            n56 = call <userlib>:"Fit VI window to Largest Dec__ogtk.vi"("error in (no error)"=w189, "border spacing (2 px)"=0) -> ("error out"=w190:errorcluster)  [unwired: 4 in, 1 out]
            n57 = call <vilib>:"Add State(s) to Queue__jki_lib_state_machine.vi"("State(s) in (\"\")"=w195) -> ("States Out"=w194:string)  [unwired: 14 in]
          }
          frame "UI: Wait" {
            # "Do not put any code in this frame.\n(It is a separator no-op. You can make a copy of this frame to create a new UI frame)"
            n58 = Scan From String(format string="%d", input string=w196, default 1=u32 0 ("default value 1")) -> (output 1=w197:u32)  [unwired: 2 in, 3 out]
            n59 = Wait (ms)(milliseconds to wait=w197) -> ()  [unwired: 1 out]
            n60 = call <vilib>:"Add State(s) to Queue__jki_lib_state_machine.vi"("State(s) in (\"\")"=w204) -> ("States Out"=w203:string)  [unwired: 14 in]
          }
          frame "UI: Cursor Set" {
            # "Argument"
            # "Initialize the User Interface, here.\n(this is called automatically, by the Macro: Init)"
            n61 = disable-structure shown="Default" {
              disable-tunnel: w207 -> [w212 w215]
              disable-tunnel: [w212 w214] -> w206
              disable-tunnel: w205 -> [_ w213]
              frame condition #0 {
              }
              frame condition #1 (active) {
                n62 = case shown="\"Idle\", Default" w213 {
                  tunnel: w215 -> [w217 w219]
                  tunnel: [w216 w218] -> w214
                  frame "Idle", Default {
                    n63 = call <vilib>:"Unset Busy.vi"("error in (no error)"=w217) -> ("error out"=w216:errorcluster)  [unwired: 10 in]
                  }
                  frame "Busy" {
                    n64 = call <vilib>:"Set Busy.vi"("error in (no error)"=w219) -> ("error out"=w218:errorcluster)  [unwired: 9 in, 1 out]
                  }
                }
              }
            }
            n65 = call <vilib>:"Add State(s) to Queue__jki_lib_state_machine.vi"("State(s) in (\"\")"=w211) -> ("States Out"=w210:string)  [unwired: 14 in]
          }
          frame "UI: Front Panel State" {
            # "Argument"
            # "Set Front Panel Open or Closed\n(Usage: \"UI: Front Panel State >> Open|Close\")"
            n66 = Unbundle By Name(w223) -> ("Core.Current VI Reference"=w222:refnum<vi>)
            n67 = disable-structure shown="TARGET_TYPE==RT" {
              disable-tunnel: w225 -> [w231 w254]
              disable-tunnel: [w230 w254] -> w224
              disable-tunnel: w222 -> [w229 _]
              disable-tunnel: w221 -> [w228 _]
              frame condition #0 (active) {
                n68 = case shown="\"Close\"" w228 {
                  tunnel: w231 -> [w235 w248]
                  tunnel: [w237 w249] -> w230
                  tunnel: w229 -> [w236 w246]
                  frame "Open", Default {
                    n69 = property class="VI"(reference=w236, error in=w235) -> (reference out=w233:refnum<vi>, error out=w234:errorcluster, "FP.State"=w232:T6)
                    n70 = case shown="\"Closed\"" w232 {
                      tunnel: [w240 w243] -> w237
                      tunnel: w234 -> [w239 w243]
                      tunnel: w233 -> [w238 _]
                      frame "Closed" {
                        n71 = invoke class="VI" method="FP.Open"(reference=w238, error in=w239, "Activate"=TRUE, "State"=T6."Standard") -> (error out=w240:errorcluster)  [unwired: 1 in, 4 out]
                      }
                      frame Default {
                      }
                    }
                  }
                  frame "Close" {
                    n72 = property class="VI"(reference=w246, error in=w248) -> (reference out=w245:refnum<vi>, error out=w247:errorcluster, "FP.State"=w244:T6)
                    n73 = case shown="Default" w244 {
                      tunnel: [w250 w253] -> w249
                      tunnel: w247 -> [w250 w252]
                      tunnel: w245 -> [_ w251]
                      frame "Invalid", "Closed" {
                      }
                      frame Default {
                        n74 = invoke class="VI" method="FP.Close"(reference=w251, error in=w252) -> (error out=w253:errorcluster)  [unwired: 1 in, 2 out]
                      }
                    }
                  }
                }
              }
              frame condition #1 {
              }
            }
            n75 = call <vilib>:"Add State(s) to Queue__jki_lib_state_machine.vi"("State(s) in (\"\")"=w227) -> ("States Out"=w226:string)  [unwired: 14 in]
          }
          frame "---------- Macro ----------" {
            # "Do not put any code in this frame.\n(It is a separator no-op. You can make a copy of this frame to create a new Macro frame)"
            n76 = call <vilib>:"Add State(s) to Queue__jki_lib_state_machine.vi"("State(s) in (\"\")"=w259) -> ("States Out"=w258:string)  [unwired: 14 in]
          }
          frame "Macro: Initialize" {
            # "Initialization Macro\n(This is called once, when the VI starts)"
            n77 = call <vilib>:"Add State(s) to Queue__jki_lib_state_machine.vi"("State(s) in Front (\"\")"="Data: Initialize\nInitialize Core Data\nEvents: Register", "State(s) in (\"\")"="Process: Sync", "State(s) at Back (\"\")"="UI: Initialize\nUI: Front Panel State >> Close\nInstrument: Open\nMacro: Debug") -> ("States Out"=w263:string)  [unwired: 12 in]
            n78 = call <vilib>:"Add State(s) to Queue__jki_lib_state_machine.vi"("State(s) in Front (\"\")"=w263, "State(s) in (\"\")"=w268) -> ("States Out"=w267:string)  [unwired: 13 in]
          }
          frame "Macro: Post Error Handling" {
            # "Clear Last Error?"
            n79 = Unbundle By Name(w270) -> ("Core.Last Error.remaining states"=w272:string, "Core.Shutdown?"=w273:bool)
            n80 = Unbundle By Name(w270) -> ("Core.Last Error.error"=w276:errorcluster)
            n81 = case shown="False" FALSE {
              tunnel: w276 -> [w284 _]
              tunnel: [w284 _] -> w275
              frame False {
              }
              frame True {
              }
            }
            n82 = case shown="False" w273 {
              tunnel: w272 -> [w281 w283]
              tunnel: [w281 w282] -> w269
              frame False {
                # "These are the remaining states (at the moment the error occured). States can be altered according to business logic."
                # "NOT SHUTTING DOWN"
              }
              frame True {
                # "Developer can decide to alter the states but should be aware that during the shutdown process, there are certain states that must be run for the SMO to properly shut itself (and this process) down. As such, one can add states to perform additional clean-ups, but should append the remaining state to be executed."
                # "SHUTTING DOWN"
                n83 = call <vilib>:"Add State(s) to Queue__jki_lib_state_machine.vi"("State(s) in (\"\")"=w283) -> ("States Out"=w282:string)  [unwired: 14 in]
              }
            }
            n84 = Bundle By Name(cluster=w270, "Core.Last Error.error"=w275) -> (w271:T9)
            n85 = call <vilib>:"Add State(s) to Queue__jki_lib_state_machine.vi"("State(s) in Front (\"\")"=w269, "State(s) in (\"\")"=w280) -> ("States Out"=w279:string)  [unwired: 13 in]
          }
          frame "Macro: Run Sequence" {
            # "0,1,2,3,4,"
            # "5"
            # "Do not put any code in this frame.\n(It is a separator no-op. You can make a copy of this frame to create a new Macro frame)"
            n86 = Unbundle By Name(w291) -> ("sequence"=w287:string[], "Running Step"=w285:i32)
            n87 = Array Size(array=w287) -> (size(s)=w297:i32)
            n88 = Index Array(array=w287, index=w285) -> (element=w286:string)
            n89 = Greater Or Equal?(x=w297, y=w285) -> (x >= y?=w289:bool)
            n90 = Select(t=-1 ("Running Step"), s=w289, f=w285) -> (s? t:f=w296:i32)
            n91 = Bundle By Name(cluster=w291, "Running Step"=w296) -> (w292:T9)
            n92 = Select(t="Sequence: Status >> ...", s=w289, f="Idle //Check Event Structure\nMacro: Run Sequence" ("State(s) at Back (\"\")")) -> (s? t:f=w288:string)
            n93 = call <vilib>:"Add State(s) to Queue__jki_lib_state_machine.vi"("State(s) in Front (\"\")"=w286, "State(s) at Back (\"\")"=w288) -> ("States Out"=w290:string)  [unwired: 13 in]
            n94 = call <vilib>:"Add State(s) to Queue__jki_lib_state_machine.vi"("State(s) in Front (\"\")"=w290, "State(s) in (\"\")"=w301) -> ("States Out"=w300:string)  [unwired: 13 in]
          }
          frame "Macro: Debug" {
            # "exe?"
            # "If pane is an EXE, then close it when we exit"
            # "Macro: Debug\n(get debug behavior, determine UI and determine shutdown behavior)"
            n95 = Unbundle By Name(w305) -> ("Core.Close Panel on Exit?"=w308:bool, "SelfRef"=w313:refnum<class "Inst.Transport.lvclass">)
            n96 = property class="App"() -> ("App.Kind"=w311:T5)  [unwired: 2 in, 2 out]
            n97 = Equal?(x=w311, y=T5."Run Time System" ("Application:Kind")) -> (x = y?=w307:bool)
            n98 = call <userlib>:"Get Debug Mode.vi"("error in (no error)"=w303, "SMO"=w313) -> ("error out"=w304:errorcluster, "Behavior"=w312:T11)  [unwired: 7 in, 1 out]
            n99 = case shown="\"Normal\", Default" w312 {
              tunnel: [w317 w319] -> w309
              tunnel: w308 -> [w317 _]
              tunnel: w307 -> [_ w321]
              tunnel: [_ "UI: Front Panel State >> Open\nUI: Wait >> 1000"] -> w302
              frame "Normal", Default {
                # "respect core.close"
              }
              frame "Debug" {
                # "keep panel open\nunless exe"
                n100 = Or(x=w321, y=FALSE) -> (x .or. y?=w319:bool)
              }
            }
            n101 = Bundle By Name(cluster=w305, "Core.Close Panel on Exit?"=w309) -> (w306:T9)
            n102 = call <vilib>:"Add State(s) to Queue__jki_lib_state_machine.vi"("State(s) in Front (\"\")"=w302, "State(s) in (\"\")"=w316) -> ("States Out"=w315:string)  [unwired: 13 in]
          }
          frame "Macro: Exit" {
            # "Exit Macro\n(This is called once, when the VI exits)"
            n103 = Unbundle By Name(w323) -> ("Core.Close Panel on Exit?"=w336:bool)
            n104 = Select(t="UI: Front Panel State >> Close", s=w336, f="" ("Empty String Constant")) -> (s? t:f=w334:string)
            n105 = Bundle By Name(cluster=w323, "Core.Shutdown?"=TRUE) -> (w324:T9)
            n106 = call <vilib>:"Add State(s) to Queue__jki_lib_state_machine.vi"("State(s) in Front (\"\")"="Data: Cleanup\nEvents: Unregister", "State(s) in (\"\")"="Process: Sync", "State(s) at Back (\"\")"="Exit") -> ("States Out"=w329:string)  [unwired: 12 in]
            n107 = call <vilib>:"Add State(s) to Queue__jki_lib_state_machine.vi"("State(s) in Front (\"\")"="Instrument: Close", "State(s) in (\"\")"=w334, "State(s) at Back (\"\")"=w329) -> ("States Out"=w333:string)  [unwired: 12 in]
            n108 = call <vilib>:"Add State(s) to Queue__jki_lib_state_machine.vi"("State(s) in Front (\"\")"=w333, "State(s) in (\"\")"=w338) -> ("States Out"=w337:string)  [unwired: 13 in]
          }
          frame "---------- Process ----------" {
            # "Template Separator\n(You can make a copy of, or modify, this frame)"
            n109 = call <vilib>:"Add State(s) to Queue__jki_lib_state_machine.vi"("State(s) in (\"\")"=w343) -> ("States Out"=w342:string)  [unwired: 14 in]
          }
          frame "Process: Sync" {
            n110 = Unbundle By Name(w351) -> ("SelfRef"=w347:refnum<class "Inst.Transport.lvclass">)
            n111 = call <vilib>:"WaitOnProcessSync.vi"("error in (no error)"=w346, "SMO"=w347) -> ("error out"=w345:errorcluster, "Don't run?"=w350:bool)  [unwired: 7 in, 1 out]
            n112 = Select(t="Data: Cleanup\nEvents: Unregister\nExit", s=w350, f="" ("Empty String Constant")) -> (s? t:f=w344:string)
            n113 = call <vilib>:"Add State(s) to Queue__jki_lib_state_machine.vi"("State(s) in Front (\"\")"=w344, "State(s) in (\"\")"=w354) -> ("States Out"=w353:string)  [unwired: 13 in]
          }
          frame "---------- Events ----------" {
            # "Template Separator\n(You can make a copy of, or modify, this frame)"
            n114 = call <vilib>:"Add State(s) to Queue__jki_lib_state_machine.vi"("State(s) in (\"\")"=w359) -> ("States Out"=w358:string)  [unwired: 14 in]
          }
          frame "Events: Register" {
            n115 = Unbundle By Name(w365) -> ("SelfRef"=w366:refnum<class "Inst.Transport.lvclass">)
            n116 = call <vilib>:"GetProtectedEvents.vi"("SMO"=w366) -> ("error out"=w364:errorcluster, "SMO Protected Events"=w369:T12, "SMO out"=w363:refnum<class "Inst.Transport.lvclass">)  [unwired: 8 in]
            n117 = call "Inst.Transport.GetPrivateEvents.vi"("Instrument.Transport in"=w363) -> ("error out"=w360:errorcluster, "Transport Private Events"=w361:cluster{"MessageToProcess":refnum<user-event>})  [unwired: 8 in, 1 out]
            n118 = register-events(w369, w361) -> (reference out=w370:refnum<event-registration>, error out=w367:errorcluster)  [unwired: 2 in]
            n119 = Merge Errors(w367, w360, w364, w362) -> (w368:errorcluster)
            n120 = call <vilib>:"Add State(s) to Queue__jki_lib_state_machine.vi"("State(s) in (\"\")"=w372) -> ("States Out"=w371:string)  [unwired: 14 in]
          }
          frame "Events: Unregister" {
            n121 = Unregister For Events(event registration refnum=w375, error in=w374) -> (error out=w373:errorcluster)
            n122 = call <vilib>:"Clear Errors.vi"("error in (no error)"=w373) -> ()  [unwired: 5 in, 2 out]
            n123 = call <vilib>:"Add State(s) to Queue__jki_lib_state_machine.vi"("State(s) in (\"\")"=w378) -> ("States Out"=w377:string)  [unwired: 14 in]
          }
          frame "---------- Instrument ----------" {
            n124 = Unbundle By Name(w381) -> ("SelfRef"=w379:refnum<class "Inst.Transport.lvclass">, "HAL"=w380:refnum<class "HAL.lvclass">)
            n125 = Bundle By Name(cluster=w381, "SelfRef"=w379, "HAL"=w380) -> (w382:T9)
            n126 = call <vilib>:"Add State(s) to Queue__jki_lib_state_machine.vi"("State(s) in (\"\")"=w386) -> ("States Out"=w385:string)  [unwired: 14 in]
          }
          frame "Instrument: Open" {
            n127 = Unbundle By Name(w391) -> ("SelfRef"=w389:refnum<class "Inst.Transport.lvclass">)
            n128 = call-dynamic "Open Hardware.vi"("error in (no error)"=w390, "Instrument in"=w389) -> ("error out"=w387:errorcluster, "Instrument out"=w388:refnum<class "Inst.Transport.lvclass">)  [unwired: 8 in]
            n129 = Bundle By Name(cluster=w391, "SelfRef"=w388) -> (w392:T9)
            n130 = call <vilib>:"Add State(s) to Queue__jki_lib_state_machine.vi"("State(s) in (\"\")"=w395) -> ("States Out"=w394:string)  [unwired: 14 in]
          }
          frame "Instrument: Write" {
            n131 = Unbundle By Name(w400) -> ("SelfRef"=w397:refnum<class "Inst.Transport.lvclass">)
            n132 = call-dynamic "Write Hardware.vi"("error in (no error)"=w398, "Instrument in"=w397) -> ("error out"=w399:errorcluster, "Instrument out"=w396:refnum<class "Inst.Transport.lvclass">)  [unwired: 8 in]
            n133 = Bundle By Name(cluster=w400, "SelfRef"=w396) -> (w401:T9)
            n134 = call <vilib>:"Add State(s) to Queue__jki_lib_state_machine.vi"("State(s) in (\"\")"=w404) -> ("States Out"=w403:string)  [unwired: 14 in]
          }
          frame "Instrument: Read" {
            n135 = Unbundle By Name(w410) -> ("SelfRef"=w406:refnum<class "Inst.Transport.lvclass">)
            n136 = call-dynamic "Read Hardware.vi"("error in (no error)"=w408, "Instrument in"=w406) -> ("error out"=w409:errorcluster, "response"=w407:string, "Instrument out"=w405:refnum<class "Inst.Transport.lvclass">)  [unwired: 7 in]
            n137 = Bundle By Name(cluster=w410, "SelfRef"=w405, "MessageToProcess.Message.Data"=w407) -> (w411:T9)
            n138 = call <vilib>:"Add State(s) to Queue__jki_lib_state_machine.vi"("State(s) in (\"\")"=w414) -> ("States Out"=w413:string)  [unwired: 14 in]
          }
          frame "Instrument: Close" {
            n139 = Unbundle By Name(w419) -> ("SelfRef"=w416:refnum<class "Inst.Transport.lvclass">)
            n140 = call-dynamic "Close Hardware.vi"("error in (no error)"=w417, "Instrument in"=w416) -> ("error out"=w418:errorcluster, "Instrument out"=w415:refnum<class "Inst.Transport.lvclass">)  [unwired: 8 in]
            n141 = Bundle By Name(cluster=w419, "SelfRef"=w415) -> (w420:T9)
            n142 = call <vilib>:"Add State(s) to Queue__jki_lib_state_machine.vi"("State(s) in (\"\")"=w423) -> ("States Out"=w422:string)  [unwired: 14 in]
          }
          frame "Instrument: Do Something" {
            # "communicate with\nhardware"
            n143 = Unbundle By Name(w431) -> ("SelfRef"=w430:refnum<class "Inst.Transport.lvclass">, "MessageToProcess.Message.Data"=w428:variant, "MessageToProcess.Message.ID"=w425:string)
            n144 = Empty String/Path?(string/path=w428) -> (empty?=w424:bool)
            n145 = case shown="False" w424 {
              tunnel: w430 -> [w440 w442]
              tunnel: [w437 w442] -> w427
              tunnel: [w436 w441] -> w426
              tunnel: w428 -> [w439 _]
              tunnel: w429 -> [w438 w441]
              tunnel: w425 -> [_ _]
              frame False {
                # "send data to\ninstrument:process.vi"
                n146 = call <userlib>:"setAllData.vi"("error in (no error)"=w438, "AllData"=w439, "Instrument in"=w440) -> ("error out"=w436:errorcluster, "Instrument out"=w437:refnum<class "Inst.Transport.lvclass">)  [unwired: 7 in]
              }
              frame True {
              }
            }
            n147 = Bundle By Name(cluster=w431, "SelfRef"=w427) -> (w432:T9)
            n148 = call <vilib>:"Add State(s) to Queue__jki_lib_state_machine.vi"("State(s) in (\"\")"=w435) -> ("States Out"=w434:string)  [unwired: 14 in]
          }
          frame "Instrument: Log" {
            # "THIS process.vi is responsible for logging data. Logging can be triggered in the timeout (as shown in this template proces.vi's tieout case) OR it could be triggered by data changes, or any other way you can device.\n\nThe code above will log ALL data. But you have the ability to log a subset, log some items on a different schedule, etc."
            n149 = Unbundle By Name(w451) -> ("SelfRef"=w447:refnum<class "Inst.Transport.lvclass">)
            n150 = call-dynamic "Get SMO Database Paths.vi"("error in (no error)"=w444, "Instrument.Transport in"=w447) -> ("error out"=w445:errorcluster, "Paths"=w448:string, "Instrument.Transport out"=w443:refnum<class "Inst.Transport.lvclass">)  [unwired: 7 in]
            n151 = Unbundle By Name(w443) -> ("Data"=w446:T13)
            n152 = call <userlib>:"Instrument.logToDatabase.vi"("error in (no error)"=w445, "Data"=w446, "Paths"=w448, "Instrument"=w443) -> ("error out"=w449:errorcluster, "Instrument out"=w450:refnum<class "Inst.Transport.lvclass">)  [unwired: 6 in]
            n153 = Bundle By Name(cluster=w451, "SelfRef"=w450) -> (w452:T9)
            n154 = call <vilib>:"Add State(s) to Queue__jki_lib_state_machine.vi"("State(s) in (\"\")"=w455) -> ("States Out"=w454:string)  [unwired: 14 in]
          }
          frame "---------- Sequence ----------" {
            n155 = call <vilib>:"Add State(s) to Queue__jki_lib_state_machine.vi"("State(s) in (\"\")"=w460) -> ("States Out"=w459:string)  [unwired: 14 in]
          }
          frame "Sequence: Status" {
            # "Sequence: Status\n(Use this frame to pass the status to the UI, this VI's UI, etc)"
            n156 = call <vilib>:"Add State(s) to Queue__jki_lib_state_machine.vi"("State(s) in (\"\")"=w466) -> ("States Out"=w465:string)  [unwired: 14 in]
            "Status" <- w461
          }
          frame "Sequence: Wait" {
            # "Sequence: Wait\n(Non-Blocking Wait)"
            # "F = repeat this state. wait\nT = go to next state. don't wait"
            n157 = Unbundle By Name(w475) -> ("Running Step"=w468:i32)
            n158 = call <userlib>:"Wait Logic.vi"("error in (no error)"=w471, "Time"=w469) -> ("error out"=w470:errorcluster, "Status String"=w467:string, "Trigger"=w472:bool)  [unwired: 6 in, 1 out]
            n159 = Increment(x=w468) -> (x+1=w482:i32)
            n160 = Select(t=w482, s=w472, f=w468) -> (s? t:f=w473:i32)
            n161 = Select(t=u32 0, s=w472, f=u32 100 ("milliseconds to wait")) -> (s? t:f=w479:u32)
            n162 = call <userlib>:"Wait (ms)__ogtk.vi"("error in (no error)"=w470, "milliseconds to wait"=w479) -> ("error out"=w477:errorcluster)  [unwired: 8 in, 1 out]
            n163 = Bundle By Name(cluster=w475, "Running Step"=w473) -> (w474:T9)
            n164 = call <vilib>:"Build State String with Arguments__JKI_lib_State_Machine.vi"("Arguments (\"\")"=w467, "State"="Sequence: Status") -> ("State with Arguments"=w476:string)  [unwired: 4 in]
            n165 = call <vilib>:"Add State(s) to Queue__jki_lib_state_machine.vi"("State(s) in Front (\"\")"=w476, "State(s) in (\"\")"=w485) -> ("States Out"=w484:string)  [unwired: 13 in]
          }
        }
      }
    }
    frame Error {
    }
  }
  n166 = case shown="No Error" w37 {
    selector: w37 -> [w496 w549]
    tunnel: w36 -> [w499 _]
    tunnel: [w492 w549] -> w35
    frame No Error {
      w489 = 0.0  # Command
      # "Can be replace with\nuse of Private Event"
      n167 = Create User Event(user event datatype=w489) -> (user event=w488:refnum<user-event>)  [unwired: 1 in, 1 out]
      n168 = call <vilib>:"GetProtectedEvents.vi"("error in (no error)"=w496, "SMO"=w499) -> ("error out"=w497:errorcluster, "SMO Protected Events"=w500:T12, "SMO out"=w498:refnum<class "Inst.Transport.lvclass">)  [unwired: 7 in]
      n169 = register-events(w500, w488) -> (reference out=w490:refnum<event-registration>)  [unwired: 2 in, 1 out]
      n170 = call <vilib>:"WaitOnProcessSync.vi"("error in (no error)"=w497, "SMO"=w498) -> ("error out"=w494:errorcluster, "Don't run?"=w493:bool, "SMO out"=w495:refnum<class "Inst.Transport.lvclass">)  [unwired: 7 in]
      n171 = case shown="False" w493 {
        tunnel: w494 -> [w505 w547]
        tunnel: w495 -> [w506 _]
        tunnel: w490 -> [w511 w548]
        tunnel: [w503 w547] -> w492
        tunnel: [w510 w548] -> w491
        tunnel: [w504 w546] -> w487
        tunnel: w488 -> [w504 w546]
        frame False {
          w513 = i64 50  # Period (ms)
          # "Destroy if created here"
          # "Destroy notifier\nto stop timed loop"
          # "Comm channel\nbetween loops\n(Can be replaced by\nclass member methods)"
          # "Sync Process\non Stop"
          n172 = Obtain Notifier(notification data type=0.0 ("Setpoint")) -> (notifier out=w507:refnum<notifier>)  [unwired: 3 in, 2 out]
          n173 = node-c288(w513) -> (w515:T14)  [unwired: 3 in]
          n174 = while {
            tunnel: w511 -> [w521]
            tunnel: [w520] -> w510
            tunnel: [w517] -> w509
            tunnel: w507 -> [w518]
            tunnel: w506 -> [w516]
            stop <- w519 stop-if-true
            # "Event Loop - HANDLING INCOMING MESSAGES"
            n175 = event shown="[1] <Command>: User Event" {
              selector: w521 -> [_ _ _ _]
              dyn-events: [_ _ _ _] -> w520
              timeout: -1 -> [_ _ _ _]
              tunnel: [_ w525 TRUE TRUE] -> w519
              tunnel: w518 -> [w523 w529 w530 w532]
              tunnel: [w523 w528 w530 w532] -> w517
              tunnel: w516 -> [_ _ _ _]
              event Timeout {
                n176 = event-data() -> ()  [unwired: 1 in, 1 out]
              }
              event User Event {
                # "Handle Command"
                n177 = event-data() -> ("Command"=w527:dbl)  [unwired: 1 in]
                n178 = Send Notification(notification=w527, notifier=w529) -> (notifier out=w528:refnum<notifier>, error out=w526:errorcluster)  [unwired: 1 in]
                n179 = Compound Arithmetic op=OR(w526, FALSE) -> (w525:bool)
              }
              event User Event {
                # "Stop SMO"
                n180 = event-data() -> ()  [unwired: 1 in, 1 out]
              }
              event User Event {
                # "Abort SMO"
                n181 = event-data() -> ()  [unwired: 1 in, 1 out]
              }
            }
          }
          n182 = timed-loop {
            timing: w515 -> [_]
            timing-out: [_] -> w514
            tunnel: w507 -> [w539]
            shift-right: [w536] -> w512
            shift-left: w506 -> [w536]
            shift-right: [w535] -> w501
            shift-left: w505 -> [w535]
            stop <- w537 stop-if-true
            # "Do\nAction"
            # "Perform \nCalculations"
            # "Get Latest\nValue"
            # "Control Loop - STATE MACHINE"
            n183 = node-c288() -> ()  [unwired: 1 in, 1 out]
            n184 = Get Notifier Status(notifier=w539) -> (current notification=w534:dbl, error out=w538:errorcluster)  [unwired: 1 in, 3 out]
            n185 = Increment(x=w534) -> ()  [unwired: 1 out]
            n186 = node-c288() -> ()  [unwired: 1 in, 1 out]
            n187 = Compound Arithmetic op=OR(w535, w538) -> (w537:bool)
          }
          n188 = node-c288(w514) -> ()  [unwired: 1 out]
          n189 = Release Notifier(notifier=w509) -> ()  [unwired: 2 in, 3 out]
          n190 = call <vilib>:"WaitOnProcessSync.vi"("SMO"=w512) -> ("error out"=w502:errorcluster)  [unwired: 8 in, 2 out]
          n191 = Merge Errors(w501, w502) -> (w503:errorcluster)
        }
        frame True {
        }
      }
      n192 = Unregister For Events(event registration refnum=w491) -> ()  [unwired: 1 in, 1 out]
      n193 = Destroy User Event(user event=w487) -> ()  [unwired: 1 in, 1 out]
    }
    frame Error {
    }
  }
  n194 = call-parent "Process.vi"("error in"=w33, "Instrument"=w40) -> ("error out"=w39:errorcluster)  [unwired: 8 in, 1 out]
  n195 = call-parent "Process.vi"("error in"=w37, "Instrument"=w36) -> ("error out"=w34:errorcluster, "Instrument out"=→"Instrument.Transport out":refnum<class "Inst.Transport.lvclass">)  [unwired: 8 in]
  n196 = Index Array(array=string[] []) -> (element #1=w16:string, element #2=w10:string, element #3=w9:string, element #4=w8:string)  [unwired: 4 in]
  "Calling VI" <- w16
  "Experiment Folder" <- w10
  "Comments" <- w9
  n197 = call "extract_tdms_params.vi"("Input String"=w8) -> ("Output Array"=w6:cluster{"key":string, "value":dbl}[])
  "TDMS Params" <- w6
  n198 = call <userlib>:"Control Experiment FGV.vi"("Function"=enum16{"read", "write"}."read", "Control Experiment.lvclass"=refnum<class "Control Experiment.lvclass"> refnum) -> ("error out"=w12:errorcluster, "Control Experiment.lvclass out"=w14:refnum<class "Control Experiment.lvclass">)  [unwired: 8 in]
  n199 = call <userlib>:"Write Experiment Folder.vi"("error in (no error)"=w12, "Experiment Folder"=w10, "Control Experiment in"=w14) -> ("error out"=w11:errorcluster, "Control Experiment out"=w13:refnum<class "Control Experiment.lvclass">)  [unwired: 7 in]
  n200 = call <userlib>:"Write Experiment Description.vi"("error in (no error)"=w11, "Experiment Description"=w9, "Control Experiment in"=w13) -> ("Control Experiment out"=w7:refnum<class "Control Experiment.lvclass">)  [unwired: 7 in, 1 out]
  n201 = call <userlib>:"Write Dictionary Elements (Loop).vi"("Data in"=w6, "Control Experiment in"=w7) -> ("Control Experiment out"=w5:refnum<class "Control Experiment.lvclass">)  [unwired: 8 in, 1 out]
  n202 = Merge Errors(w34, w35) -> ()  [unwired: 1 out]
  n203 = Merge Errors(w39, w38) -> (→"error out":errorcluster)
  n204 = call <userlib>:"Write Dependencies.vi"("Control Experiment"=w5, "Transport in"=w2) -> ("Transport out"=w20:refnum<class "Transport.lvclass">)  [unwired: 8 in, 1 out]
  n205 = Create User Event(user event datatype=w2) -> (user event=w1:refnum<user-event>)  [unwired: 1 in, 1 out]
  n206 = Obtain Notifier(notification data type=w2) -> ()  [unwired: 3 in, 3 out]
  n207 = Obtain Notifier(notification data type=FALSE) -> (notifier out=w18:refnum<notifier>, error out=w22:errorcluster)  [unwired: 3 in, 1 out]
  n208 = register-events(w1) -> ()  [unwired: 3 in, 2 out]
  n209 = call <userlib>:"Write notifier.vi"("error in (no error)"=w22, "notifier"=w18, "Transport in"=w20) -> ("error out"=w24:errorcluster, "Transport out"=w26:refnum<class "Transport.lvclass">)  [unwired: 7 in]
  n210 = call <userlib>:"Write Configure Sweep.vi"("error in (no error)"=w24, "Lockin_Sweep"=T1 {"Sweep Time (s)"=0.0, "Initial Wait (s)"=0.0, "Return to Start"=FALSE, "Sweep Channels"=[], "Sweep Tables"=[]}, "Transport in"=w26) -> ("error out"=w23:errorcluster, "Transport out"=w25:refnum<class "Transport.lvclass">)  [unwired: 7 in]
  n211 = while {
    tunnel: w18 -> [w552]
    tunnel: [w554] -> _
    tunnel: [w553] -> w30
    stop <- "stop" stop-if-true
    # "Loop that sends notifications"
    n212 = Send Notification(notification="stop 2", notifier=w552) -> (notifier out=w554:refnum<notifier>, error out=w553:errorcluster)  [unwired: 1 in]
  }
  n213 = while {
    tunnel: w18 -> [w562]
    tunnel: [w563] -> w29
    tunnel: w25 -> [w561]
    tunnel: w23 -> [w560]
    tunnel: w22 -> [w559]
    tunnel: [w556] -> w19
    tunnel: w16 -> [w555]
    stop <- w566 stop-if-true
    # "This loop will repeat until a stop notification is received"
    # "Loop that listens to notifications"
    n214 = case shown="\"Lockin_sweep\"" w555 {
      tunnel: w561 -> [w569 _ w573 w576]
      tunnel: w560 -> [w568 w570 w572 w575]
      tunnel: [w567 w570 w571 w574] -> w558
      frame "Lockin_sweep" {
        n215 = call <userlib>:"Lockin_sweep.vi"("Transport"=w569, "error in (no error)"=w568) -> ("error out"=w567:errorcluster)  [unwired: 7 in, 1 out]
      }
      frame Default {
      }
      frame "Lockin_time" {
        n216 = call <userlib>:"Lockin_time.vi"("error in (no error)"=w572, "Transport"=w573) -> ("error out"=w571:errorcluster)  [unwired: 8 in, 1 out]
      }
      frame "THz_TimeDelay" {
        n217 = call <userlib>:"THz_TimeDelay.vi"("error in (no error)"=w575, "Transport"=w576) -> ("error out"=w574:errorcluster)  [unwired: 8 in, 1 out]
      }
    }
    n218 = Merge Errors(w558, w559) -> (w557:errorcluster)
    n219 = Get Notifier Status(notifier=w562, error in (no error)=w557) -> (notifier out=w556:refnum<notifier>, current notification=w565:bool, error out=w564:errorcluster)  [unwired: 2 out]
    n220 = Or(x=w565, y=w564) -> (x .or. y?=w566:bool)
    n221 = call <vilib>:"Clear Errors.vi"("error in (no error)"=w564) -> ("error out"=w563:errorcluster)  [unwired: 5 in, 1 out]
  }
  n222 = Merge Errors(w30, w29) -> (w28:errorcluster)
  n223 = Release Notifier(notifier=w19, force destroy? (F)=TRUE, error in (no error)=w28) -> ()  [unwired: 3 out]
